vi "Start Acquisition.vi"(8 "error in (no error)":errorcluster, 10 "Continuous":bool, 11 "Data Source in":refnum<class "Data Source.lvclass">) -> (0 "error out":errorcluster, 3 "Data Source out":refnum<class "Data Source.lvclass">)   [LabVIEW 2020, in "Data Source.lvlib" / "Data Source.lvclass"]
uses:
  Data Source.lvclass
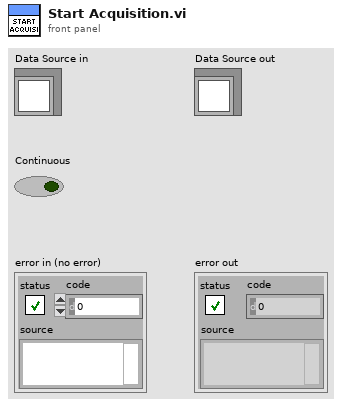
[diagram p1: front panel]
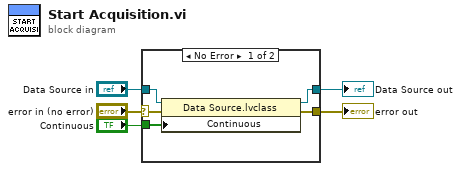
[diagram p0: block diagram]
diagram:
  n1 = case shown="No Error" "error in (no error)" {
    selector: "error in (no error)" -> [w8 w12]
    tunnel: [w7 w12] -> w4
    tunnel: [w9 w11] -> w2
    tunnel: "Data Source in" -> [w10 w11]
    tunnel: "Continuous" -> [w6 _]
    frame No Error {
      n2 = property class="Data Source.lvclass"(reference=w10, error in=w8, "Continuous"=w6) -> (reference out=w9:refnum<class "Data Source.lvclass">, error out=w7:errorcluster)
    }
    frame Error {
    }
  }
  "error out" <- w4
  "Data Source out" <- w2
